vi "Time and Date.vi"(0 "VISA resource name":refnum<visa-resource-name>, 7 "Time and Date Value":timestamp format="%<%H:%M:%S\n%Y/%m/%d>T", 11 "error in (no error)":errorcluster) -> (4 "VISA resource name out":refnum<visa-resource-name>, 15 "error out":errorcluster)   [LabVIEW 2020, in "Keithley 27XX.lvlib"]
doc: "Use this VI to set the current Time and Date on your instrument."
uses:
  <instrlib>/Keithley 27XX/Keithley 27XX.lvlib
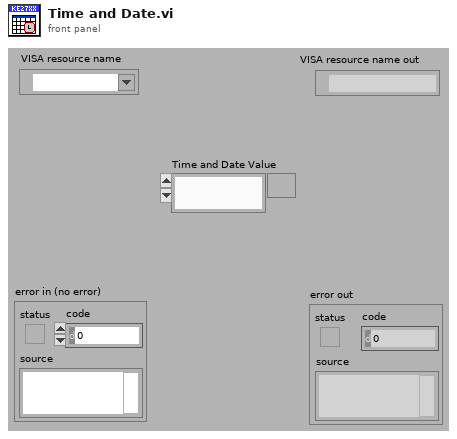
[diagram p1: front panel]
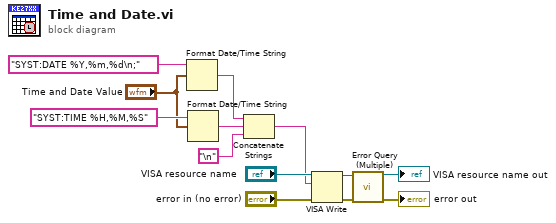
[diagram p0: block diagram]
diagram:
  n1 = Format Date/Time String(time format string (%c)="SYST:DATE %Y,%m,%d\n;", seconds (now)="Time and Date Value") -> (date/time string=w3:string)  [unwired: 1 in]
  n2 = Format Date/Time String(time format string (%c)="SYST:TIME %H,%M,%S", seconds (now)="Time and Date Value") -> (date/time string=w2:string)  [unwired: 1 in]
  n3 = Concatenate Strings(w3, w2, "\n") -> (w6:string)
  n4 = VISA Write(VISA resource name="VISA resource name", write buffer=w6, error in (no error)="error in (no error)") -> (VISA resource name out=w8:refnum<visa-resource-name>, error out=w7:errorcluster)  [unwired: 1 out]
  n5 = call <instrlib>:"Error Query (Multiple).vi"("VISA resource name"=w8, "error in (no error)"=w7) -> ("VISA resource name out"=→"VISA resource name out":refnum<visa-resource-name>, "error out"=→"error out":errorcluster)  [unwired: 10 in, 2 out]
